vi "Generate Documentation from VIs.vi"(0 "search dir":path=path "C:/ADIBitbucket/nists19.0_templateproject/Code Modules/Common/Instrument Control/DCPower", 5 "output file path":path=path "C:/Users/marobert/Desktop/STSDevToolsDocProj/documentation/DCPower.md", 7 "dir filter":T1, 9 "image dir":path=path "C:/Users/marobert/Desktop/STSDevToolsDocProj/documentation/images", 11 "error in":errorcluster) -> (4 "Report":string, 6 "Number of Folders":i32, 8 "Number of Files":i32, 15 "error out":errorcluster)   [LabVIEW 2019, in "MD Generator.lvlib"]
uses:
  MD Generator.lvlib
  Filter.ctl
  <userlib>/_OpenG.lib/array/array.llb/Search 1D Array (Path)__ogtk.vi
  <userlib>/_OpenG.lib/array/array.llb/Index 1D Array Elements (Path)__ogtk.vi
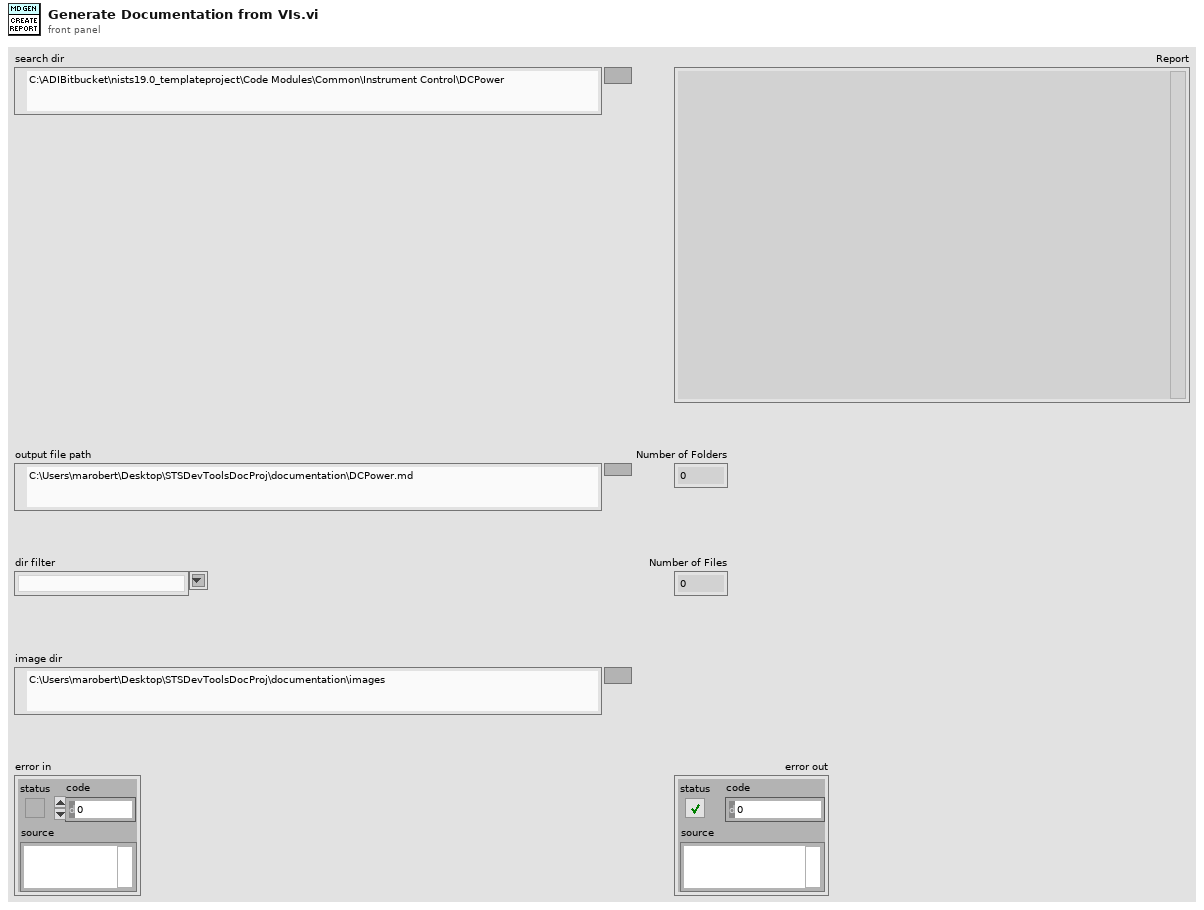
[diagram p1: front panel]
types:
  T1 = typedef "MD Generator.lvlib/Filter.ctl" = string
  T2 = enum16{"open", "replace", "create", "open or create", "replace or create", "replace or create with confirmation"}
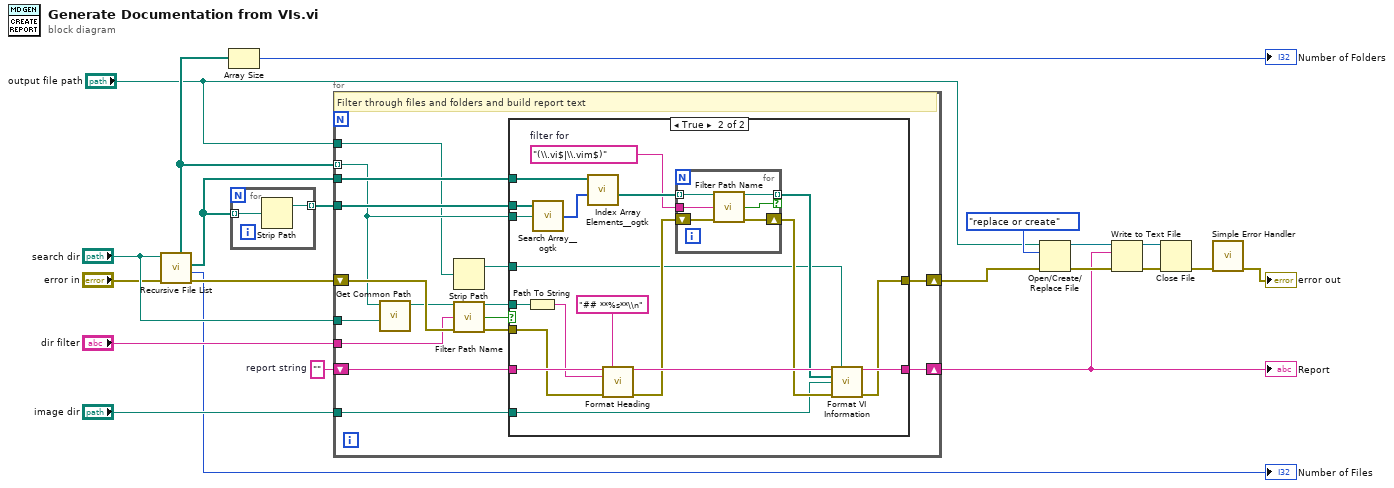
[diagram p0: block diagram]
diagram:
  w13 = ""  # report string
  n1 = call <vilib>:"Recursive File List.vi"("error in (no error)"="error in", "Folder Path"="search dir") -> ("error out"=w14:errorcluster, "Number of Files"=→"Number of Files":i32, "All Files in Dir"=w15:path[], "All Folders"=w19:path[])  [unwired: 5 in, 1 out]
  n2 = Array Size(array=w19) -> (size(s)=→"Number of Folders":i32)
  n3 = for {
    tunnel: w15 -> [w23] mode=indexing
    tunnel: [w22] -> w18 mode=indexing
    n4 = Strip Path(path=w23) -> (stripped path=w22:path)  [unwired: 1 out]
  }
  n5 = for {
    tunnel: w19 -> [w25] mode=indexing
    tunnel: "search dir" -> [w27]
    tunnel: w18 -> [w38]
    tunnel: w15 -> [w37]
    shift-right: [w35] -> w4
    shift-left: w13 -> [w36]
    shift-right: [w34] -> w5
    shift-left: w14 -> [w39]
    tunnel: "dir filter" -> [w32]
    tunnel: "image dir" -> [w28]
    tunnel: "output file path" -> [w24]
    # "Filter through files and folders and build report text"
    n6 = call "Get Common Path.vi"("Root Path"=w27, "Target Path"=w25) -> ("Relative Path"=w33:path)  [unwired: 8 in, 1 out]
    n7 = Strip Path(path=w24) -> (stripped path=w26:path)  [unwired: 1 out]
    n8 = call "Filter Path Name.vi"("file or directory paths"=w33, "filter for"=w32, "error in"=w39) -> ("matched file paths"=w29:path, "matched"=w30:bool, "error out"=w31:errorcluster)  [unwired: 10 in]
    n9 = case shown="True" w30 {
      tunnel: w38 -> [_ w59]
      tunnel: w25 -> [_ w45]
      tunnel: w37 -> [_ w58]
      tunnel: w36 -> [w40 w56]
      tunnel: [w40 w55] -> w35
      tunnel: [w41 w54] -> w34
      tunnel: w31 -> [w41 w53]
      tunnel: w29 -> [_ w52]
      tunnel: w28 -> [_ w43]
      tunnel: w26 -> [_ w42]
      frame False {
      }
      frame True {
        w44 = T1 "(\\.vi$|\\.vim$)"  # filter for
        n10 = Path To String(path=w52) -> (string=w47:string)
        n11 = call-poly <userlib>:"Search Array__ogtk.vi"("Array"=w59, "Element Data"=w45) -> ("Indices of Elements"=w60:i32[])  [unwired: 7 in]
        n12 = call-poly <userlib>:"Index Array Elements__ogtk.vi"("indices"=w60, "array"=w58) -> ("elements"=w51:path[])  [unwired: 9 in]
        n13 = call "Format Heading.vi"("string In"=w56, "format string"="## **%s**\\n" ("heading format string"), "new heading"=w47, "error in"=w53) -> ("string out"=w57:string, "error out"=w50:errorcluster)  [unwired: 10 in]
        n14 = for {
          tunnel: w51 -> [w66] mode=indexing
          tunnel: [w65] -> w48 mode=indexing if=w64
          shift-right: [w63] -> w49
          shift-left: w50 -> [w62]
          tunnel: w44 -> [w61]
          n15 = call "Filter Path Name.vi"("file or directory paths"=w66, "filter for"=w61, "error in"=w62) -> ("matched file paths"=w65:path, "matched"=w64:bool, "error out"=w63:errorcluster)  [unwired: 10 in]
        }
        n16 = call "Format VI Information.vi"("string in"=w57, "output dir"=w42, "file paths"=w48, "image dir"=w43, "error in"=w49) -> ("string out"=w55:string, "error out"=w54:errorcluster)  [unwired: 9 in]
      }
    }
  }
  "Report" <- w4
  n17 = Open/Create/Replace File(file path (use dialog)="output file path", error in=w5, operation (0:open)=T2."replace or create") -> (refnum out=w11:refnum<file>, error out=w10:errorcluster)  [unwired: 3 in, 1 out]
  n18 = Write to Text File(file (use dialog)=w11, text=w4, error in=w10) -> (refnum out=w9:refnum<file>, error out=w8:errorcluster)  [unwired: 1 in, 1 out]
  n19 = Close File(refnum=w9, error in=w8) -> (error out=w6:errorcluster)  [unwired: 1 out]
  n20 = call <vilib>:"Simple Error Handler.vi"("error in (no error)"=w6) -> ("error out"=→"error out":errorcluster)  [unwired: 4 in, 4 out]
